vi "AnalyzePulseTrain CBC Fix.vi"(0 "Waveform In":waveform(dbl)={"t0"=timestamp(3433165898.5470004 s since 1904-01-01), "dt"=1e-05, "Y"=array[4250 elements]}, 5 "Repetitions in the Input Waveform":i32, 7 "Pulse Characteristics":T1={"Pulses per Cycle"=2, "Load Resistance (Ohms)"=750.0, "Krec Value"=2, "Recovery Mode (T=Active)"=TRUE, "Target Stim Currents (Amps)"=[]} {"Target Stim Currents (Amps)" format="%#_6p"}) -> (2 "Avg. CBC Width":dbl format="%0.6f", 3 "Avg. CBC Amplitude":dbl format="%0.2f", 4 "Stim PW":dbl[](array[numeric]), 6 "Stim Amplitude":dbl[](array[numeric]), 8 "Interphase Delay":dbl[](array[numeric]), 10 "Recovery PW":dbl[](array[numeric]), 12 "Waveform Parameters":T2 {"Frequency" format="%#_6p"; "Avg CBC Width" format="%#_6p"; "Avg. CBC Holdoff" format="%#_6p"; "Stim Pulse Width" format="%^#_6g"; "Interphase Delay" format="%#_6p"; "Recovery PW" format="%#_6p"; "Recovery Holdoff" format="%#_6p"; "Stim Amplitude" format="%^#_6g"; "Recovery Amplitude" format="%#_6p"}, 13 "Frequency":dbl, 14 "Recovery Holdoff":dbl[](array[numeric]), 15 "Recovery Amplitude":dbl[](array[numeric]))   [LabVIEW 2010]
uses:
  <vilib>/measure/mamon.llb/Trigger Detection for 1 Channel.vi
  <vilib>/measure/NI_MAPro.lvlib
  <vilib>/Analysis/NI_AALBase.lvlib
panel:
  in  "View":enum32{"View All", "Graph Only"}(tab)
  out "Waveform in ( graph )":waveform(dbl)(graph)
  out "Normalized Waveform":waveform(dbl)(graph)
  out "Offset":dbl
  out "Eq. Freq ( Hz )":dbl format="%#_6p"
  out "Current in amps":waveform(dbl)(graph)
  out "Time2 - Time1 ( sec )":dbl format="%#_6p"
  out "index":i32
  # "Remove idle voltage offset\n( if applicable )"
  # "The input waveform should be a capture of the STIM chip output\n(before the cap) when the output is held at 1/2 HVDD by the\nLoad Resistance.  This ensures that passive recovery and CBC\npulses are captured, because they look like pulses pulled to GND."
  # "The elements in these arrays correspond to the pulses per cycle.\nThey are the averages over all the repetitions in the waveform."
  # "Enter Target Current\nfor each in array below"
  # "1. Update Cursor Positions\n2. Turn off X Autoscaling\n3. Run this VI again"
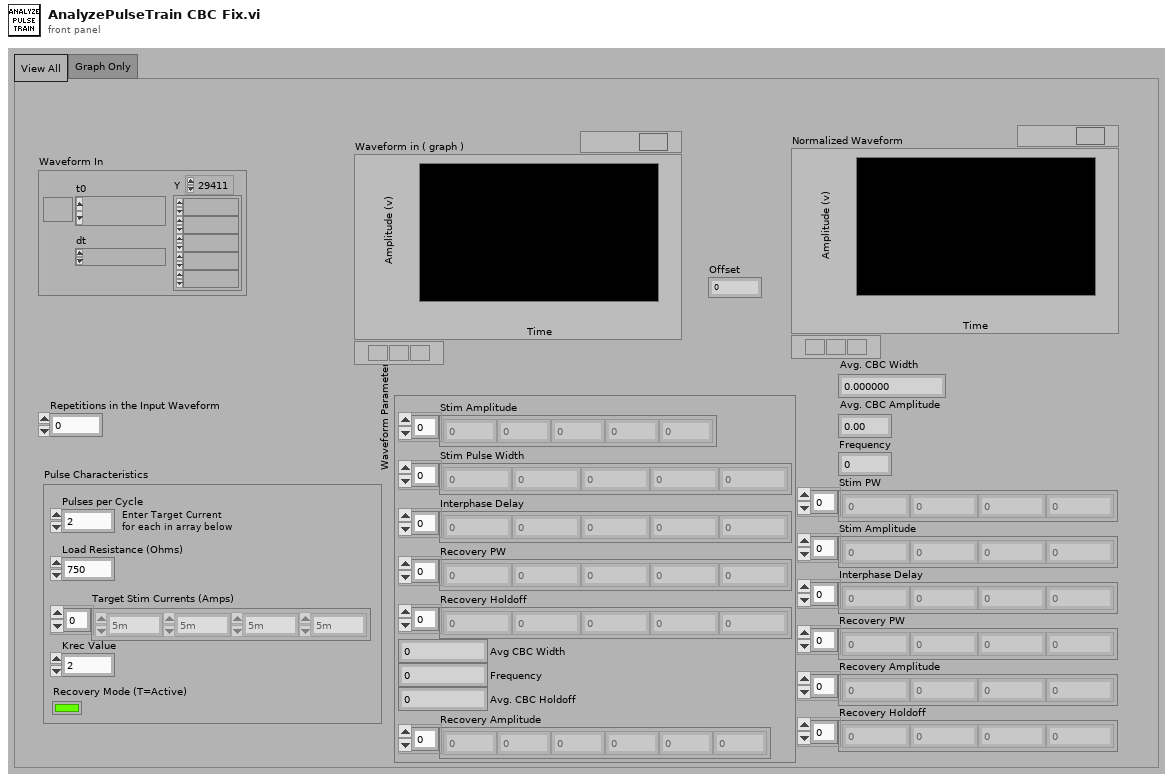
[diagram p1: front panel]
types:
  T1 = cluster{"Pulses per Cycle":i32, "Load Resistance (Ohms)":dbl, "Krec Value":i32, "Recovery Mode (T=Active)":bool, "Target Stim Currents (Amps)":dbl[]}
  T2 = cluster{"Stim Amplitude":dbl[], "Stim Pulse Width":dbl[], "Interphase Delay":dbl[], "Recovery PW":dbl[], "Recovery Holdoff":dbl[], "Avg CBC Width":dbl, "Frequency":dbl, "Avg. CBC Holdoff":dbl, "Recovery Amplitude":dbl[]}
  T3 = cluster{"trigger slope":u16, "Trigger Level":dbl}[]
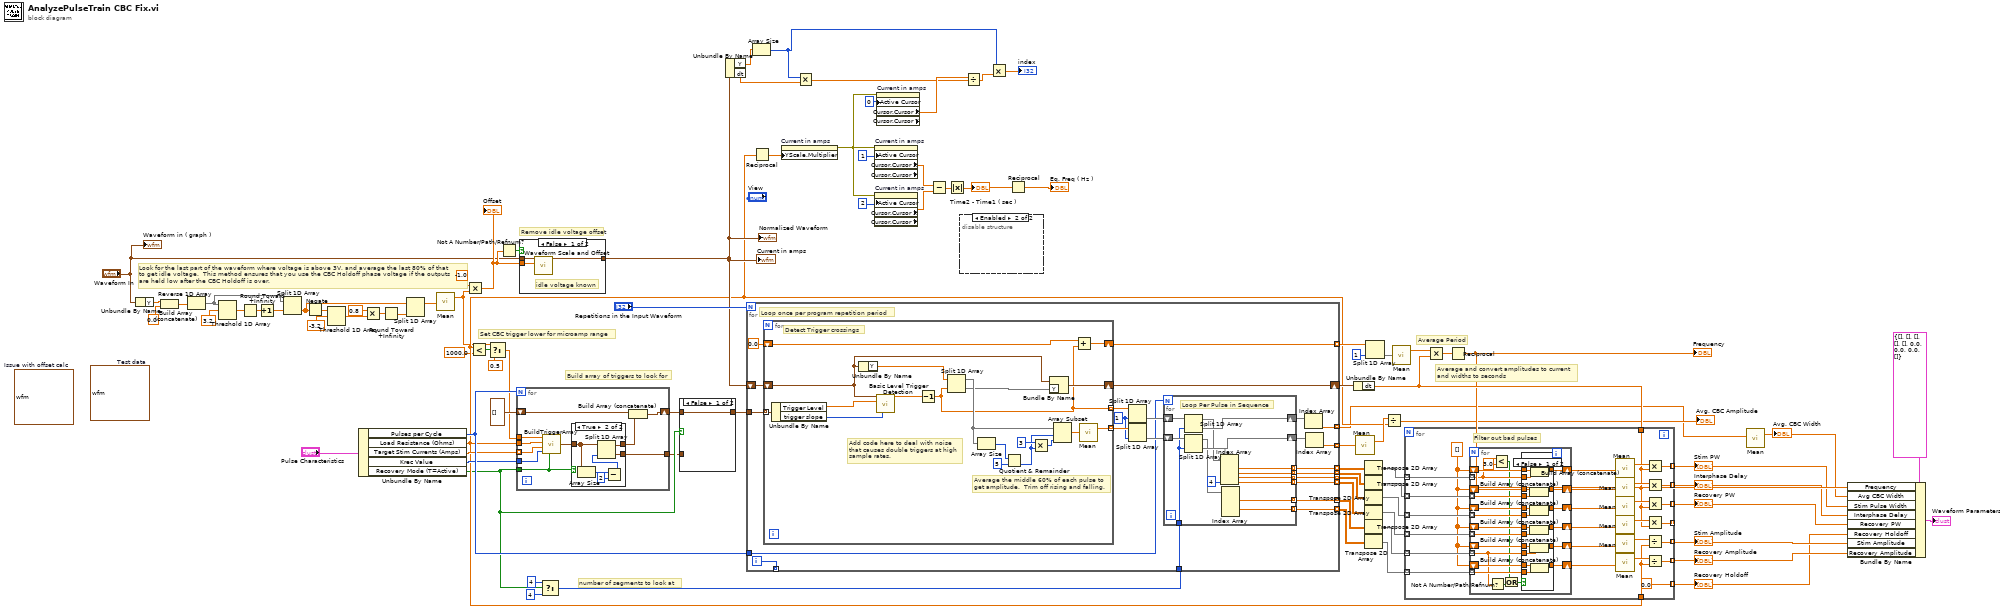
[diagram p0: block diagram]
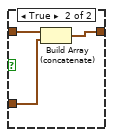
[diagram p2: hidden frame]
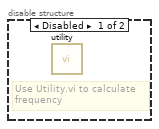
[diagram p3: hidden frame]
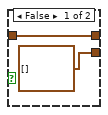
[diagram p6: hidden frame]
diagram:
  (unwired) waveform(dbl) {"t0"=timestamp(3458836317.3280005 s since 1904-01-01), "dt"=1.428e-05, "Y"=array[4000 elements]}  # Issue with offset calc
  (unwired) waveform(dbl) {"t0"=timestamp(3418839276.250478 s since 1904-01-01), "dt"=1e-06, "Y"=[5.0, 5.0, 9.0, 9.0, 9.0, 9.0, 9.0, 9.0, 9.0, 9.0, 5.0, 5.0, 5.0, 3.0, 3.0, 3.0, 3.0, 3.0, 3.0, 3.0, 3.0, 3.0, 3.0, 3.0, 3.0, 3.0, 3.0, 3.0, 3.0, 5.0, 5.0, 5.0, 5.0, 8.0, 8.0, 8.0, 8.0, 8.0, 8.0, 8.0, 8.0, 5.0, 5.0, 5.0, 3.0, 3.0, 3.0, 3.0, 3.0, 3.0, 3.0, 3.0, 3.0, 3.0, 3.0, 3.0, 3.0, 3.0, 3.0, 3.0, 5.0, 5.0, 5.0, 5.0, 0.0, 0.0, 0.0, 0.0, 0.0, 5.0, 5.0, 5.0, 5.0, 5.0, 5.0, 5.0, 5.0, 5.0, 5.0, 5.0, 5.0, 5.0, 5.0, 5.0, 5.0, 5.0, 5.0, 5.0, 5.0, 5.0, 5.0, 5.0, 5.0, 5.0, 5.0, 5.0, 5.0, 5.0, 5.0, 5.0, 5.0, 5.0, 9.0, 9.0, 9.0, 9.0, 9.0, 9.0, 9.0, 9.0, 5.0, 5.0, 5.0, 3.0, 3.0, 3.0, 3.0, 3.0, 3.0, 3.0, 3.0, 3.0, 3.0, 3.0, 3.0, 3.0, 3.0, 3.0, 3.0, 5.0, 5.0, 5.0, 5.0, 8.0, 8.0, 8.0, 8.0, 8.0, 8.0, 8.0, 8.0, 5.0, 5.0, 5.0, 3.0, 3.0, 3.0, 3.0, 3.0, 3.0, 3.0, 3.0, 3.0, 3.0, 3.0, 3.0, 3.0, 3.0, 3.0, 3.0, 5.0, 5.0, 5.0, 5.0, 0.0, 0.0, 0.0, 0.0, 0.0, 5.0, 5.0, 5.0, 5.0, 5.0, 5.0, 5.0, 5.0, 5.0, 5.0, 5.0, 5.0, 5.0, 5.0, 5.0, 5.0, 5.0, 5.0, 5.0, 5.0, 5.0, 5.0, 5.0, 5.0, 5.0, 5.0, 5.0, 5.0, 5.0, 5.0, 5.0, 5.0, 5.0, 9.0, 9.0, 9.0, 9.0, 9.0, 9.0, 9.0, 9.0, 5.0, 5.0, 5.0, 3.0, 3.0, 3.0, 3.0, 3.0, 3.0, 3.0, 3.0, 3.0, 3.0, 3.0, 3.0, 3.0, 3.0, 3.0, 3.0, 5.0, 5.0, 5.0, 5.0, 8.0, 8.0, 8.0, 8.0, 8.0, 8.0, 8.0, 8.0, 5.0, 5.0, 5.0, 3.0, 3.0, 3.0, 3.0, 3.0, 3.0, 3.0, 3.0, 3.0, 3.0, 3.0, 3.0, 3.0, 3.0, 3.0, 3.0, 5.0, 5.0, 5.0, 5.0, 0.0, 0.0, 0.0, 0.0, 0.0, 5.0, 5.0, 5.0, 5.0, 5.0, 5.0, 5.0, 5.0, 5.0, 5.0, 5.0, 5.0, 5.0, 5.0, 5.0, 5.0, 5.0, 5.0, 5.0, 5.0, 5.0, 5.0, 5.0, 5.0, 5.0, 5.0, 5.0, 5.0, 5.0, 5.0, 5.0, 5.0, 5.0, 9.0, 9.0, 9.0, 9.0, 9.0, 9.0, 9.0, 9.0, 5.0, 5.0, 5.0, 3.0, 3.0, 3.0, 3.0, 3.0, 3.0, 3.0, 3.0, 3.0, 3.0, 3.0, 3.0, 3.0, 3.0, 3.0, 3.0, 5.0, 5.0, 5.0, 5.0, 8.0, 8.0, 8.0, 8.0, 8.0, 8.0, 8.0, 8.0, 5.0, 5.0, 5.0, 3.0, 3.0, 3.0, 3.0, 3.0, 3.0, 3.0, 3.0, 3.0, 3.0, 3.0, 3.0, 3.0, 3.0, 3.0, 3.0, 5.0, 5.0, 5.0, 5.0, 0.0, 0.0, 0.0, 0.0, 0.0, 5.0, 5.0, 5.0, 5.0, 5.0, 5.0, 5.0, 5.0, 5.0, 5.0, 5.0, 5.0, 5.0, 5.0, 5.0, 5.0, 5.0, 5.0, 5.0, 5.0, 5.0, 5.0, 5.0, 5.0, 5.0, 5.0, 5.0, 5.0, 5.0, 5.0, 5.0, 5.0, 5.0, 9.0, 9.0, 9.0, 9.0, 9.0, 9.0, 9.0, 9.0, 5.0, 5.0, 5.0, 3.0, 3.0, 3.0, 3.0, 3.0, 3.0, 3.0, 3.0, 3.0, 3.0, 3.0, 3.0, 3.0, 3.0, 3.0, 3.0, 5.0, 5.0, 5.0, 5.0, 8.0, 8.0, 8.0, 8.0, 8.0, 8.0, 8.0, 8.0, 5.0, 5.0, 5.0, 3.0, 3.0, 3.0, 3.0, 3.0, 3.0, 3.0, 3.0, 3.0, 3.0, 3.0, 3.0, 3.0, 3.0, 3.0, 3.0, 5.0, 5.0, 5.0, 5.0, 0.0, 0.0, 0.0, 0.0, 0.0, 5.0, 5.0, 5.0, 5.0, 5.0, 5.0, 5.0, 5.0, 5.0, 5.0, 5.0, 5.0, 5.0, 5.0, 5.0, 5.0, 5.0, 5.0, 5.0, 5.0, 5.0, 5.0, 5.0, 5.0, 5.0, 5.0, 5.0, 5.0, 5.0, 5.0, 5.0, 5.0, 5.0, 5.0]}  # Test data
  # "Set CBC trigger lower for microamp range"
  # "number of segments to look at"
  # "Look for the last part of the waveform where voltage is above 3V, and average the last 80% of that\nto get idle voltage.  This method ensures that you use the CBC Holdoff phase voltage if the outputs\nare held low after the CBC Holdoff is over."
  # "Average Period"
  # "Average and convert amplitudes to current\nand widths to seconds"
  # "Build array of triggers to look for"
  # "Remove idle voltage offset"
  n1 = Unbundle By Name("Waveform In") -> ("Y"=w14:dbl[])
  n2 = Build Array (concatenate)(w14, 0.0 ("y")) -> (w13:dbl[])
  n3 = Reverse 1D Array(array=w13) -> (reversed array=w12:dbl[])
  n4 = Threshold 1D Array(2:3.2 ("y"), 3:w12) -> (0:w54:dbl)  [unwired: 1 in]
  n5 = Round Toward +Infinity(x=w54) -> (ceil(x): smallest int >= x=w53:dbl)
  n6 = Increment(x=w53) -> (x+1=w46:dbl)
  n7 = Split 1D Array(array=w12, index=w46) -> (second subarray=w37:dbl[])  [unwired: 1 out]
  n8 = Negate(x=w37) -> (-x=w51:dbl[])
  n9 = Threshold 1D Array(2:-3.2 ("y"), 3:w51) -> (0:w50:dbl)  [unwired: 1 in]
  n10 = Unbundle By Name("Pulse Characteristics") -> ("Pulses per Cycle"=w75:i32, "Load Resistance (Ohms)"=w11:dbl, "Target Stim Currents (Amps)"=w23:dbl[], "Krec Value"=w74:i32, "Recovery Mode (T=Active)"=w5:bool)
  n11 = Multiply(x=0.8, y=w50) -> (x*y=w48:dbl)
  n12 = Round Toward +Infinity(x=w48) -> (ceil(x): smallest int >= x=w47:dbl)
  n13 = Split 1D Array(array=w37, index=w47) -> (first subarray=w36:dbl[])  [unwired: 1 out]
  n14 = call <vilib>:"Mean.vi"("X"=w36) -> ("mean"=w8:dbl)  [unwired: 1 out]
  n15 = Multiply(x=-1.0, y=w8) -> (x*y=w39:dbl)
  "Offset" <- w39
  n16 = Less?(x=w11, y=1000.0) -> (x < y?=w9:bool)
  n17 = Select(t=w8, s=w9, f=0.5) -> (s? t:f=w7:dbl)
  n18 = Not A Number/Path/Refnum?(number/path/refnum=w39) -> (NaN/Path/Refnum?=w38:bool)
  n19 = for {
    N: w75 -> [_]
    shift-right: [w100] -> w4
    shift-left: T3 [] -> [w99]
    tunnel: w7 -> [w98]
    tunnel: w5 -> [w94]
    tunnel: w11 -> [w97]
    tunnel: w23 -> [w96] mode=indexing
    tunnel: w74 -> [w95]
    tunnel: [w91] -> w2
    n20 = call "BuildTriggerArray.vi"("CBC Trigger Level"=w98, "Load Resistance (Ohms)"=w97, "Target Stim Current (Amps)"=w96, "Krec Value"=w95, "Recovery Mode (T=Active)"=w94) -> ("Pulse Triggers"=w93:T3)
    n21 = case shown="True" w94 {
      tunnel: w93 -> [w102 w106]
      tunnel: [w102 w108] -> w92
      tunnel: [T3 [] w107] -> w91
      frame False {
      }
      frame True {
        n22 = Array Size(array=w106) -> (size(s)=w105:i32)
        n23 = Subtract(x=w105, y=2) -> (x-y=w103:i32)
        n24 = Split 1D Array(array=w106, index=w103) -> (first subarray=w108:T3, second subarray=w107:T3)
      }
    }
    n25 = Build Array (concatenate)(w99, w92) -> (w100:T3)
  }
  n26 = case shown="False" w38 {
    tunnel: [w111 w112] -> w22
    tunnel: "Waveform In" -> [w110 w112]
    tunnel: w39 -> [w109 _]
    frame False {
      # "idle voltage known"
      n27 = call <vilib>:"Waveform Scale and Offset.vi"("offset"=w109, "waveform in"=w110) -> ("waveform out"=w111:waveform(dbl))  [unwired: 8 in, 1 out]
    }
    frame True {
      # "Unknown Idle Voltage"
    }
  }
  "Normalized Waveform" <- w22
  "Current in amps" <- w22
  n28 = Select(t=4, s=w5, f=4 ("index")) -> (s? t:f=w42:i32)
  n29 = case shown="False" w5 {
    tunnel: w4 -> [w113 w116]
    tunnel: [w113 w115] -> w3
    tunnel: w2 -> [_ w114]
    frame False {
    }
    frame True {
      n30 = Build Array (concatenate)(w116, w114) -> (w115:T3)
    }
  }
  n31 = Unbundle By Name(w22) -> ("Y"=w18:dbl[], "dt"=w17:dbl)
  n32 = for {
    N: "Repetitions in the Input Waveform" -> [_]
    tunnel: w3 -> [w139]
    shift-right: [w135] -> w72
    shift-left: w22 -> [w138]
    tunnel: w75 -> [w132]
    tunnel: [w129] -> w1 mode=indexing
    tunnel: [w128] -> w88 mode=indexing
    tunnel: [w127] -> w87 mode=indexing
    tunnel: [w126] -> w86 mode=indexing
    tunnel: [w125] -> w85 mode=indexing
    tunnel: [w124] -> w84 mode=indexing
    tunnel: [w123] -> w83 mode=indexing
    tunnel: [w122] -> w82 mode=indexing
    tunnel: [w119] -> w70 mode=indexing
    tunnel: w42 -> [w118]
    tunnel: [w117] -> _ mode=indexing
    i -> [w117]
    w136 = 1 ("index")
    # "Loop once per program repetition period"
    n33 = for {
      tunnel: w139 -> [w172] mode=indexing
      shift-right: [w159] -> w135
      shift-left: w138 -> [w155]
      tunnel: [w164] -> w137 mode=indexing
      tunnel: [w157] -> w120 mode=indexing
      shift-right: [w163] -> w119
      shift-left: 0.0 -> [w162]
      # "Add code here to deal with noise \nthat causes double triggers at high\nsample rates."
      # "Detect Trigger crossings"
      # "Average the middle 60% of each pulse to\nget amplitude.  Trim off rising and falling."
      n34 = Unbundle By Name(w172) -> ("Trigger Level"=w161:dbl, "trigger slope"=w160:u16)
      n35 = Unbundle By Name(w155) -> ("Y"=w156:dbl[])
      n36 = call-poly <vilib>:"Basic Level Trigger Detection.vi"("signal in"=w155, "level"=w161, "trigger slope"=w160) -> ("trigger location"=w154:dbl)  [unwired: 10 in, 2 out]
      n37 = Decrement(x=w154) -> (x-1=w157:dbl)
      n38 = Split 1D Array(array=w156, index=w157) -> (first subarray=w166:dbl[], second subarray=w158:dbl[])
      n39 = Array Size(array=w166) -> (size(s)=w171:i32)
      n40 = Quotient & Remainder(x=w171, y=5) -> (floor(x/y)=w168:i32)  [unwired: 1 out]
      n41 = Multiply(x=3, y=w168) -> (x*y=w167:i32)
      n42 = Bundle By Name(cluster=w155, "Y"=w158) -> (w159:waveform(dbl))
      n43 = Array Subset(array=w166, index=w168, length=w167) -> (w165:dbl[])
      n44 = Add(x=w162, y=w157) -> (x+y=w163:dbl)
      n45 = call <vilib>:"Mean.vi"("X"=w165) -> ("mean"=w164:dbl)  [unwired: 1 out]
    }
    n46 = Split 1D Array(array=w120, index=w136) -> (second subarray=w134:dbl[])  [unwired: 1 out]
    n47 = Split 1D Array(array=w137, index=w136) -> (second subarray=w133:dbl[])  [unwired: 1 out]
    n48 = for {
      N: w132 -> [_]
      shift-right: [w151] -> w131
      shift-left: w134 -> [w153]
      shift-right: [w150] -> w130
      shift-left: w133 -> [w152]
      tunnel: [w147] -> w127 mode=indexing
      tunnel: [w146] -> w126 mode=indexing
      tunnel: [w145] -> w125 mode=indexing
      tunnel: [w144] -> w124 mode=indexing
      tunnel: [w143] -> w123 mode=indexing
      tunnel: [w142] -> w122 mode=indexing
      tunnel: w118 -> [w141]
      # "Loop Per Pulse in Sequence"
      n49 = Split 1D Array(array=w153, index=w141) -> (first subarray=w149:dbl[], second subarray=w151:dbl[])
      n50 = Split 1D Array(array=w152, index=w141) -> (first subarray=w148:dbl[], second subarray=w150:dbl[])
      n51 = Index Array(array=w149, index #4=4 ("index")) -> (element #1=w147:dbl, element #2=w146:dbl, element #3=w145:dbl, element #4=w144:dbl)  [unwired: 3 in]
      n52 = Index Array(array=w148) -> (element #1=w143:dbl, element #3=w142:dbl)  [unwired: 4 in, 2 out]
    }
    n53 = Index Array(array=w131) -> (element=w129:dbl)  [unwired: 1 in]
    n54 = Index Array(array=w130) -> (element=w128:dbl)  [unwired: 1 in]
  }
  n55 = Array Size(array=w18) -> (size(s)=w16:i32)
  n56 = Reciprocal(x=w11) -> (1/x=w40:dbl)
  n57 = property on="Current in amps" class="WFGraph (strict)"("YScale.Multiplier"=w40) -> (error out=w25:errorcluster)  [unwired: 2 in, 1 out]
  n58 = Multiply(x=w16, y=w17) -> (x*y=w15:dbl)
  n59 = property on="Current in amps" class="WFGraph (strict)" props=["Active Cursor", "Cursor", "Cursor X", "Cursor", "Cursor Y"](error in=w25, "Active Cursor"=u32 1) -> ("Cursor.Cursor X"=w29:dbl)  [unwired: 1 in, 3 out]
  n60 = property on="Current in amps" class="WFGraph (strict)" props=["Active Cursor", "Cursor", "Cursor X", "Cursor", "Cursor Y"](error in=w25, "Active Cursor"=u32 2) -> ("Cursor.Cursor X"=w28:dbl)  [unwired: 1 in, 3 out]
  n61 = property on="Current in amps" class="WFGraph (strict)" props=["Active Cursor", "Cursor", "Cursor X", "Cursor", "Cursor Y"](error in=w25, "Active Cursor"=u32 0) -> ("Cursor.Cursor X"=w21:dbl)  [unwired: 1 in, 3 out]
  n62 = Subtract(x=w29, y=w28) -> (x-y=w30:dbl)
  n63 = Absolute Value(x=w30) -> (abs(x)=w27:dbl)
  "Time2 - Time1 ( sec )" <- w27
  n64 = disable-structure shown="Enabled" {
    frame Disabled {
      # "Use Utility.vi to calculate\nfrequency"
      n65 = call "utility.vi"() -> ()  [unwired: 12 in]
    }
    frame Enabled {
    }
  }
  n66 = Divide(x=w21, y=w15) -> (x/y=w20:dbl)
  n67 = Multiply(x=w16, y=w20) -> (x*y=→"index":dbl)
  n68 = Reciprocal(x=w27) -> (1/x=→"Eq. Freq ( Hz )":dbl)
  n69 = Unbundle By Name(w72) -> ("dt"=w67:dbl)
  n70 = call <vilib>:"Mean.vi"("X"=w88) -> ("mean"=w71:dbl)  [unwired: 1 out]
  n71 = Transpose 2D Array(2D array=w87) -> (transposed array=w81:dbl[][])
  n72 = Transpose 2D Array(2D array=w86) -> (transposed array=w80:dbl[][])
  n73 = Transpose 2D Array(2D array=w85) -> (transposed array=w79:dbl[][])
  n74 = Transpose 2D Array(2D array=w84) -> (transposed array=w78:dbl[][])
  n75 = Transpose 2D Array(2D array=w83) -> (transposed array=w77:dbl[][])
  n76 = Transpose 2D Array(2D array=w82) -> (transposed array=w76:dbl[][])
  n77 = Split 1D Array(array=w70, index=1) -> (second subarray=w69:dbl[])  [unwired: 1 out]
  n78 = Divide(x=w71, y=w11) -> (x/y=→"Avg. CBC Amplitude":dbl)
  n79 = call <vilib>:"Mean.vi"("X"=w69) -> ("mean"=w68:dbl)  [unwired: 1 out]
  n80 = for {
    tunnel: w81 -> [w180] mode=indexing
    tunnel: w80 -> [w185] mode=indexing
    tunnel: w79 -> [w184] mode=indexing
    tunnel: w78 -> [w183] mode=indexing
    tunnel: w77 -> [w182] mode=indexing
    tunnel: w76 -> [w181] mode=indexing
    tunnel: [w200] -> w61 mode=indexing
    tunnel: [w199] -> w60 mode=indexing
    tunnel: [w198] -> w59 mode=indexing
    tunnel: [w197] -> _ mode=indexing
    tunnel: [w196] -> w58 mode=indexing
    tunnel: [w195] -> w57 mode=indexing
    tunnel: w67 -> [w188]
    tunnel: w11 -> [w187]
    tunnel: [0.0 ("Load Resistance (Ohms)")] -> w45 mode=indexing
    w179 = dbl[] []
    # "Filter out bad pulses"
    n81 = for {
      tunnel: w180 -> [w203] mode=indexing
      tunnel: w185 -> [w210] mode=indexing
      tunnel: w184 -> [w209] mode=indexing
      tunnel: w183 -> [w208] mode=indexing
      tunnel: w182 -> [w206] mode=indexing
      tunnel: w181 -> [w207] mode=indexing
      shift-right: [w221] -> w178
      shift-left: w179 -> [w222]
      shift-right: [w219] -> w177
      shift-left: w179 -> [w220]
      shift-right: [w217] -> w176
      shift-left: w179 -> [w218]
      shift-right: [w215] -> w175
      shift-left: w179 -> [w216]
      shift-right: [w213] -> w174
      shift-left: w179 -> [w214]
      shift-right: [w211] -> w173
      shift-left: w179 -> [w212]
      n82 = Not A Number/Path/Refnum?(number/path/refnum=w206) -> (NaN/Path/Refnum?=w204:bool)
      n83 = Less?(x=w203, y=3.0) -> (x < y?=w201:bool)
      n84 = Or(x=w201, y=w204) -> (x .or. y?=w205:bool)
      n85 = case shown="False" w205 {
        tunnel: w222 -> [w238 w246]
        tunnel: [w239 w246] -> w221
        tunnel: w220 -> [w227 w245]
        tunnel: [w232 w245] -> w219
        tunnel: w218 -> [w226 w244]
        tunnel: [w231 w244] -> w217
        tunnel: w216 -> [w225 w243]
        tunnel: [w230 w243] -> w215
        tunnel: w214 -> [w224 w242]
        tunnel: [w229 w242] -> w213
        tunnel: w212 -> [w223 w241]
        tunnel: [w228 w241] -> w211
        tunnel: w203 -> [w240 _]
        tunnel: w210 -> [w237 _]
        tunnel: w209 -> [w236 _]
        tunnel: w208 -> [w235 _]
        tunnel: w206 -> [w234 _]
        tunnel: w207 -> [w233 _]
        frame False {
          n86 = Build Array (concatenate)(w227, w237) -> (w232:dbl[])
          n87 = Build Array (concatenate)(w226, w236) -> (w231:dbl[])
          n88 = Build Array (concatenate)(w225, w235) -> (w230:dbl[])
          n89 = Build Array (concatenate)(w224, w234) -> (w229:dbl[])
          n90 = Build Array (concatenate)(w238, w240) -> (w239:dbl[])
          n91 = Build Array (concatenate)(w223, w233) -> (w228:dbl[])
        }
        frame True {
        }
      }
    }
    n92 = call <vilib>:"Mean.vi"("X"=w178) -> ("mean"=w193:dbl)  [unwired: 1 out]
    n93 = call <vilib>:"Mean.vi"("X"=w177) -> ("mean"=w192:dbl)  [unwired: 1 out]
    n94 = call <vilib>:"Mean.vi"("X"=w176) -> ("mean"=w191:dbl)  [unwired: 1 out]
    n95 = call <vilib>:"Mean.vi"("X"=w175) -> ("mean"=w190:dbl)  [unwired: 1 out]
    n96 = call <vilib>:"Mean.vi"("X"=w174) -> ("mean"=w189:dbl)  [unwired: 1 out]
    n97 = call <vilib>:"Mean.vi"("X"=w173) -> ("mean"=w194:dbl)  [unwired: 1 out]
    n98 = Multiply(x=w193, y=w188) -> (x*y=w200:dbl)
    n99 = Multiply(x=w192, y=w188) -> (x*y=w199:dbl)
    n100 = Multiply(x=w191, y=w188) -> (x*y=w198:dbl)
    n101 = Multiply(x=w190, y=w188) -> (x*y=w197:dbl)
    n102 = Divide(x=w189, y=w187) -> (x/y=w196:dbl)
    n103 = Divide(x=w194, y=w187) -> (x/y=w195:dbl)
  }
  "Stim PW" <- w61
  "Interphase Delay" <- w60
  "Recovery PW" <- w59
  "Recovery Holdoff" <- w45
  "Stim Amplitude" <- w58
  "Recovery Amplitude" <- w57
  n104 = Multiply(x=w68, y=w67) -> (x*y=w66:dbl)
  n105 = Reciprocal(x=w66) -> (1/x=w63:dbl)
  "Frequency" <- w63
  n106 = call <vilib>:"Mean.vi"("X"=w1) -> ("mean"=w44:dbl)  [unwired: 1 out]
  "Avg. CBC Width" <- w44
  n107 = Bundle By Name(cluster=T2 {"Stim Amplitude"=[], "Stim Pulse Width"=[], "Interphase Delay"=[], "Recovery PW"=[], "Recovery Holdoff"=[], "Avg CBC Width"=0.0, "Frequency"=0.0, "Avg. CBC Holdoff"=0.0, "Recovery Amplitude"=[]} ("Pulse Train Parameters"), "Frequency"=w63, "Avg CBC Width"=w44, "Stim Pulse Width"=w61, "Interphase Delay"=w60, "Recovery PW"=w59, "Recovery Holdoff"=w45, "Stim Amplitude"=w58, "Recovery Amplitude"=w57) -> (→"Waveform Parameters":T2)
  "Waveform in ( graph )" <- "Waveform In"
